vi "TIS_Camera_Polarimeter.vi"() -> ()   [LabVIEW 2025]
panel:
  in  "Degree Sampling":dbl=1.0
  in  "Calibrate QWP":bool
  in  "N Angles":i16=8 min=8 max=200 step=2
  in  "Measure Stokes":bool
  in  "Tab Control":T1(tab)
  in  "ICImagingControl":refnum<k7>(container)
  out "Snapped Image":T2(plugin-control)
  in  "Connect Camera":bool
  in  "Live":bool
  in  "Camera Properties":bool
  out "Camera Ready":bool
  in  "Grab Image":bool
  in  "Stop All":bool
  out "Motor Ready":bool
  in  "Backward":bool
  in  "Forward":bool
  in  "Motor Name":string="0"
  in  "Encoder Steps/º":i32=398
  in  "Jog Angle (º)":dbl=22.5 format="%#_13g"
  in  "VISA Rotatory Motor":refnum<visa-resource-name>="COM4"
  in  "Connect Motor":bool
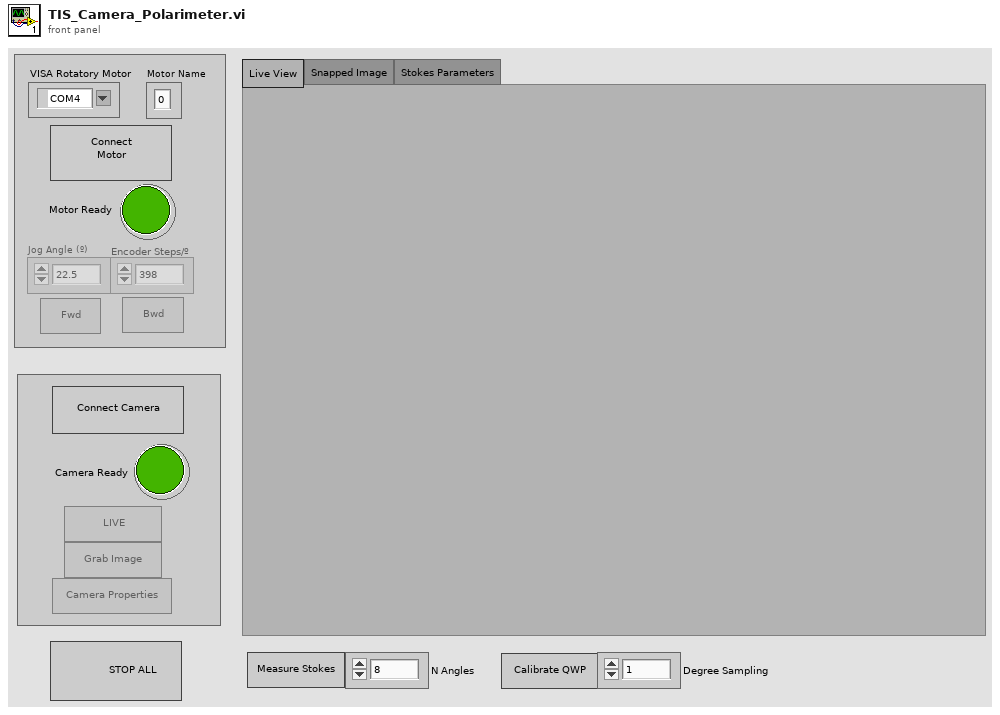
[diagram p1: front panel]
types:
  T1 = enum32{"Live View", "Snapped Image", "Stokes Parameters"}
  T2 = typedef "IMAQ Image.ctl" = refnum<image>
  T3 = typedef "Image Type" = u32
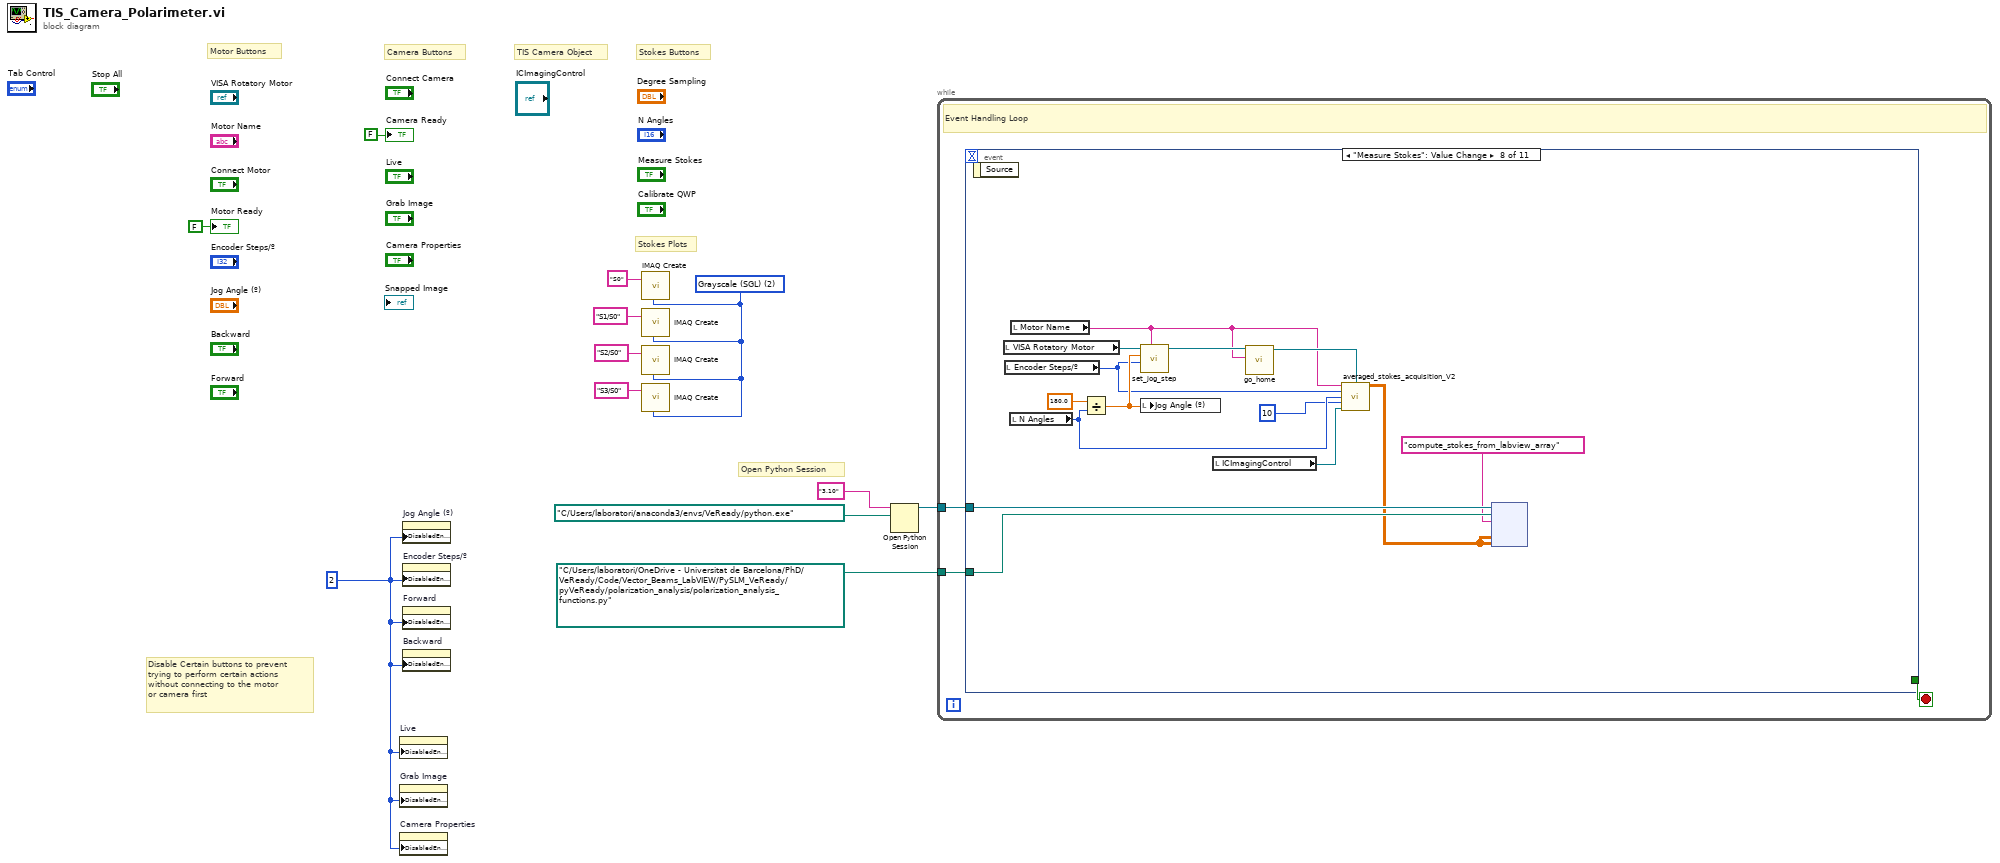
[diagram p0: block diagram]
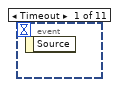
[diagram p2: hidden frame]
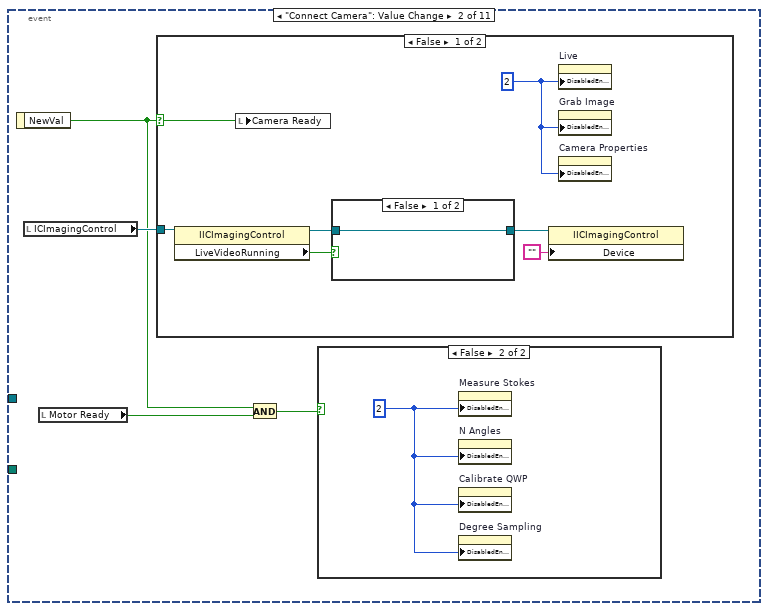
[diagram p3: hidden frame]
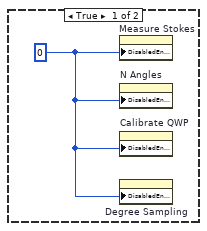
[diagram p4: hidden frame]
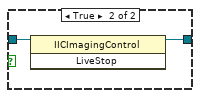
[diagram p5: hidden frame]
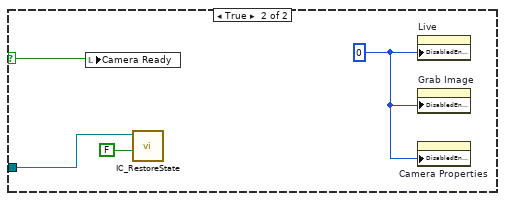
[diagram p6: hidden frame]
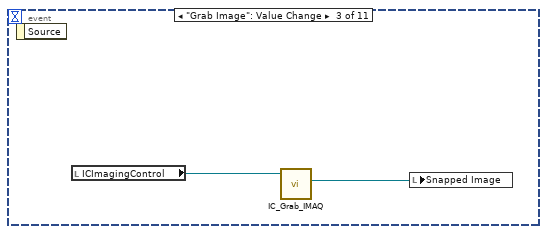
[diagram p7: hidden frame]
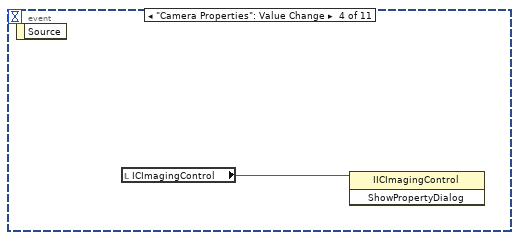
[diagram p8: hidden frame]
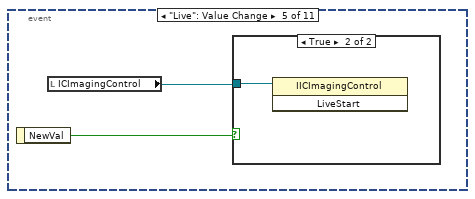
[diagram p9: hidden frame]
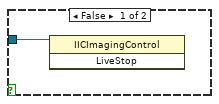
[diagram p10: hidden frame]
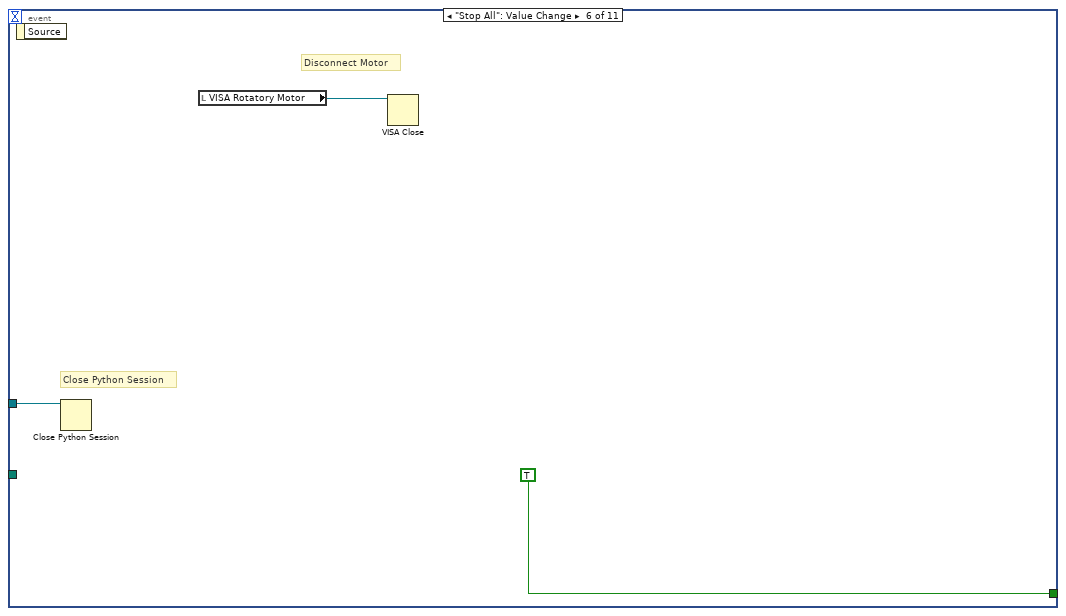
[diagram p11: hidden frame]
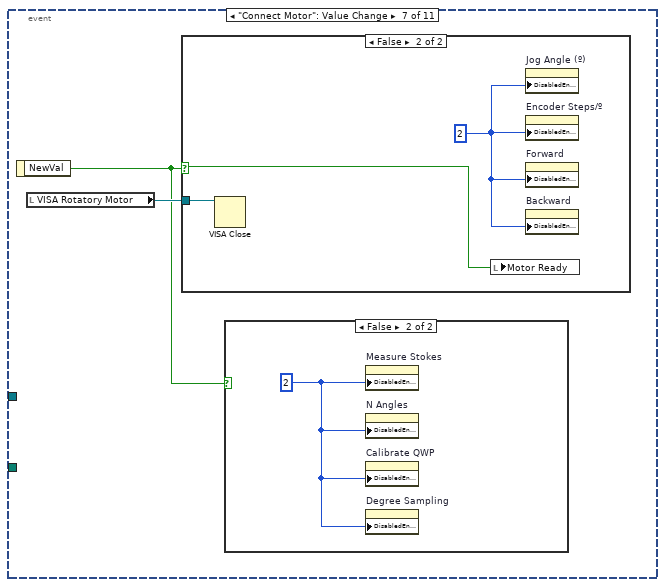
[diagram p12: hidden frame]
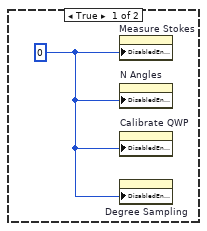
[diagram p13: hidden frame]
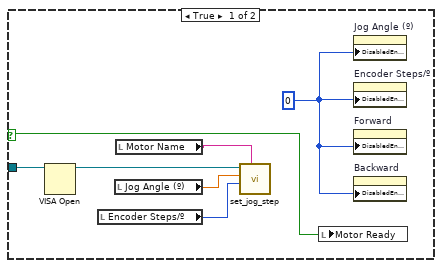
[diagram p14: hidden frame]
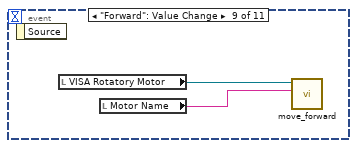
[diagram p15: hidden frame]
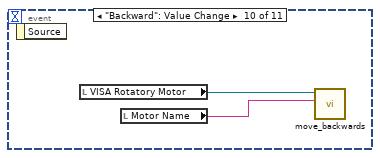
[diagram p16: hidden frame]
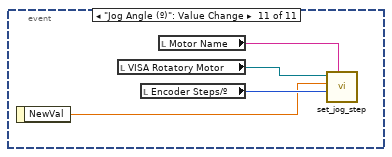
[diagram p17: hidden frame]
diagram:
  w1 = T3 2 items=["Grayscale (U8)", "Grayscale (I16)", "Grayscale (SGL)", "Complex (CSG)", "RGB (U32)", "HSL (U32)", "RGB (U64)", "Grayscale (U16)"] ("Image Type")
  w8 = 2
  # "Stokes Plots"
  # "Stokes Buttons"
  # "TIS Camera Object"
  # "Camera Buttons"
  # "Disable Certain buttons to prevent\ntrying to perform certain actions\nwithout connecting to the motor\nor camera first"
  # "Open Python Session"
  # "Motor Buttons"
  n1 = property on="Live" class="Bool (strict)"("DisabledEnum"=w8) -> ()  [unwired: 2 in, 2 out]
  n2 = property on="Grab Image" class="Bool (strict)"("DisabledEnum"=w8) -> ()  [unwired: 2 in, 2 out]
  n3 = property on="Camera Properties" class="Bool (strict)"("DisabledEnum"=w8) -> ()  [unwired: 2 in, 2 out]
  n4 = property on="Jog Angle (º)" class="DigNum (strict)"("DisabledEnum"=w8) -> ()  [unwired: 2 in, 2 out]
  n5 = property on="Encoder Steps/º" class="DigNum (strict)"("DisabledEnum"=w8) -> ()  [unwired: 2 in, 2 out]
  n6 = property on="Forward" class="Bool"("DisabledEnum"=w8) -> ()  [unwired: 2 in, 2 out]
  n7 = property on="Backward" class="Bool"("DisabledEnum"=w8) -> ()  [unwired: 2 in, 2 out]
  n8 = call "IMAQ Create"("Image Name"="S0", "Image Type"=w1) -> ()  [unwired: 3 in, 2 out]
  n9 = call "IMAQ Create"("Image Name"="S1/S0", "Image Type"=w1) -> ()  [unwired: 3 in, 2 out]
  n10 = call "IMAQ Create"("Image Name"="S2/S0", "Image Type"=w1) -> ()  [unwired: 3 in, 2 out]
  n11 = call "IMAQ Create"("Image Name"="S3/S0", "Image Type"=w1) -> ()  [unwired: 3 in, 2 out]
  n12 = Open Python Session(python version="3.10" ("Python version"), python path=path "C:/Users/laboratori/anaconda3/envs/VeReady/python.exe" ("Python path")) -> (session out=w7:refnum<k35>)  [unwired: 1 in, 1 out]
  n13 = while {
    tunnel: w7 -> [w14]
    tunnel: path "C:/Users/laboratori/OneDrive - Universitat de Barcelona/PhD/VeReady/Code/Vector_Beams_LabVIEW/PySLM_VeReady/pyVeReady/polarization_analysis/polarization_analysis_functions.py" ("module path") -> [w13]
    stop <- w15 stop-if-true
    # "Event Handling Loop"
    n14 = event shown="[7] \"Measure Stokes\": Value Change" {
      selector: _ -> [_ _ _ _ _ _ _ _ _ _ _]
      dyn-events: _ -> [_ _ _ _ _ _ _ _ _ _ _]
      timeout: _ -> [_ _ _ _ _ _ _ _ _ _ _]
      tunnel: [_ _ _ _ _ TRUE _ _ _ _ _] -> w15
      tunnel: w14 -> [_ _ _ _ _ w43 _ w63 _ _ _]
      tunnel: w13 -> [_ _ _ _ _ _ _ w62 _ _ _]
      event Timeout {
        n15 = event-data() -> ()  [unwired: 1 in, 1 out]
      }
      event "Connect Camera": Value Change {
        n16 = event-data() -> ("NewVal"=w17:bool)  [unwired: 1 in]
        n17 = local read "ICImagingControl"() -> (w19:refnum<k7>)
        n18 = local read "Motor Ready"() -> (w16:bool)
        n19 = case shown="False" w17 {
          selector: w17 -> [w22 w32]
          tunnel: w19 -> [w28 w35]
          frame False {
            w23 = 2
            n20 = property class="IICImagingControl"(reference=w28) -> (reference out=w27:refnum<k7>, "LiveVideoRunning"=w26:bool)  [unwired: 1 in, 1 out]
            n21 = local write "Camera Ready"(w22) -> ()
            n22 = case shown="False" w26 {
              tunnel: [w29 w31] -> w25
              tunnel: w27 -> [w29 w30]
              frame False {
              }
              frame True {
                n23 = invoke class="IICImagingControl" method="LiveStop"(reference=w30) -> (reference out=w31:refnum<k7>)  [unwired: 2 in, 2 out]
              }
            }
            n24 = property class="IICImagingControl"(reference=w25, "Device"="") -> ()  [unwired: 1 in, 2 out]
            n25 = property on="Live" class="Bool (strict)"("DisabledEnum"=w23) -> ()  [unwired: 2 in, 2 out]
            n26 = property on="Grab Image" class="Bool (strict)"("DisabledEnum"=w23) -> ()  [unwired: 2 in, 2 out]
            n27 = property on="Camera Properties" class="Bool (strict)"("DisabledEnum"=w23) -> ()  [unwired: 2 in, 2 out]
          }
          frame True {
            w33 = 0
            n28 = local write "Camera Ready"(w32) -> ()
            n29 = call <userlib>:"IC_RestoreState.vi"("Color"=FALSE, "ICImagingControl"=w35) -> ()  [unwired: 2 in, 2 out]
            n30 = property on="Live" class="Bool (strict)"("DisabledEnum"=w33) -> ()  [unwired: 2 in, 2 out]
            n31 = property on="Grab Image" class="Bool (strict)"("DisabledEnum"=w33) -> ()  [unwired: 2 in, 2 out]
            n32 = property on="Camera Properties" class="Bool (strict)"("DisabledEnum"=w33) -> ()  [unwired: 2 in, 2 out]
          }
        }
        n33 = And(x=w17, y=w16) -> (x .and. y?=w18:bool)
        n34 = case shown="False" w18 {
          frame True {
            w20 = 0
            n35 = property on="Measure Stokes" class="Bool (strict)"("DisabledEnum"=w20) -> ()  [unwired: 2 in, 2 out]
            n36 = property on="N Angles" class="DigNum (strict)"("DisabledEnum"=w20) -> ()  [unwired: 2 in, 2 out]
            n37 = property on="Calibrate QWP" class="Bool (strict)"("DisabledEnum"=w20) -> ()  [unwired: 2 in, 2 out]
            n38 = property on="Degree Sampling" class="DigNum (strict)"("DisabledEnum"=w20) -> ()  [unwired: 2 in, 2 out]
          }
          frame False {
            w21 = 2
            n39 = property on="Measure Stokes" class="Bool (strict)"("DisabledEnum"=w21) -> ()  [unwired: 2 in, 2 out]
            n40 = property on="N Angles" class="DigNum (strict)"("DisabledEnum"=w21) -> ()  [unwired: 2 in, 2 out]
            n41 = property on="Calibrate QWP" class="Bool (strict)"("DisabledEnum"=w21) -> ()  [unwired: 2 in, 2 out]
            n42 = property on="Degree Sampling" class="DigNum (strict)"("DisabledEnum"=w21) -> ()  [unwired: 2 in, 2 out]
          }
        }
      }
      event "Grab Image": Value Change {
        n43 = event-data() -> ()  [unwired: 1 in, 1 out]
        n44 = local read "ICImagingControl"() -> (w37:refnum<k7>)
        n45 = call <userlib>:"IC_Grab_IMAQ.vi"("ICImagingControl In"=w37) -> ("Image Out"=w36:T2)  [unwired: 2 in, 3 out]
        n46 = local write "Snapped Image"(w36) -> ()
      }
      event "Camera Properties": Value Change {
        n47 = event-data() -> ()  [unwired: 1 in, 1 out]
        n48 = local read "ICImagingControl"() -> (w38:refnum<k7>)
        n49 = invoke class="IICImagingControl" method="ShowPropertyDialog"(reference=w38) -> ()  [unwired: 2 in, 3 out]
      }
      event "Live": Value Change {
        n50 = event-data() -> ("NewVal"=w39:bool)  [unwired: 1 in]
        n51 = local read "ICImagingControl"() -> (w40:refnum<k7>)
        n52 = case shown="True" w39 {
          tunnel: w40 -> [w41 w42]
          frame False {
            n53 = invoke class="IICImagingControl" method="LiveStop"(reference=w41) -> ()  [unwired: 2 in, 3 out]
          }
          frame True {
            n54 = invoke class="IICImagingControl" method="LiveStart"(reference=w42) -> ()  [unwired: 2 in, 3 out]
          }
        }
      }
      event "Stop All": Value Change {
        # "Close Python Session"
        # "Disconnect Motor"
        n55 = event-data() -> ()  [unwired: 1 in, 1 out]
        n56 = Close Python Session(session in=w43) -> ()  [unwired: 1 in, 1 out]
        n57 = local read "VISA Rotatory Motor"() -> (w44:refnum<visa-resource-name>)
        n58 = VISA Close(VISA resource name=w44) -> ()  [unwired: 1 in, 1 out]
      }
      event "Connect Motor": Value Change {
        n59 = event-data() -> ("NewVal"=w46:bool)  [unwired: 1 in]
        n60 = local read "VISA Rotatory Motor"() -> (w47:refnum<visa-resource-name>)
        n61 = case shown="False" w46 {
          selector: w46 -> [w55 w58]
          tunnel: w47 -> [w56 w59]
          frame True {
            w54 = 0
            n62 = VISA Open(VISA resource name=w56) -> (VISA resource name=w53:refnum<visa-resource-name>)  [unwired: 4 in, 1 out]
            n63 = local read "Encoder Steps/º"() -> (w51:i32)
            n64 = local read "Jog Angle (º)"() -> (w52:dbl)
            n65 = local read "Motor Name"() -> (w50:string)
            n66 = call "set_jog_step.vi"("Motor \"Name\""=w50, "Encoder Pulses per Degree"=w51, "Degrees"=w52, "VISA resource name"=w53) -> ()  [unwired: 5 in, 2 out]
            n67 = local write "Motor Ready"(w55) -> ()
            n68 = property on="Jog Angle (º)" class="DigNum (strict)"("DisabledEnum"=w54) -> ()  [unwired: 2 in, 2 out]
            n69 = property on="Encoder Steps/º" class="DigNum (strict)"("DisabledEnum"=w54) -> ()  [unwired: 2 in, 2 out]
            n70 = property on="Forward" class="Bool"("DisabledEnum"=w54) -> ()  [unwired: 2 in, 2 out]
            n71 = property on="Backward" class="Bool"("DisabledEnum"=w54) -> ()  [unwired: 2 in, 2 out]
          }
          frame False {
            w57 = 2
            n72 = VISA Close(VISA resource name=w59) -> ()  [unwired: 1 in, 1 out]
            n73 = local write "Motor Ready"(w58) -> ()
            n74 = property on="Jog Angle (º)" class="DigNum (strict)"("DisabledEnum"=w57) -> ()  [unwired: 2 in, 2 out]
            n75 = property on="Encoder Steps/º" class="DigNum (strict)"("DisabledEnum"=w57) -> ()  [unwired: 2 in, 2 out]
            n76 = property on="Forward" class="Bool"("DisabledEnum"=w57) -> ()  [unwired: 2 in, 2 out]
            n77 = property on="Backward" class="Bool"("DisabledEnum"=w57) -> ()  [unwired: 2 in, 2 out]
          }
        }
        n78 = case shown="False" w46 {
          frame True {
            w48 = 0
            n79 = property on="Measure Stokes" class="Bool (strict)"("DisabledEnum"=w48) -> ()  [unwired: 2 in, 2 out]
            n80 = property on="N Angles" class="DigNum (strict)"("DisabledEnum"=w48) -> ()  [unwired: 2 in, 2 out]
            n81 = property on="Calibrate QWP" class="Bool (strict)"("DisabledEnum"=w48) -> ()  [unwired: 2 in, 2 out]
            n82 = property on="Degree Sampling" class="DigNum (strict)"("DisabledEnum"=w48) -> ()  [unwired: 2 in, 2 out]
          }
          frame False {
            w49 = 2
            n83 = property on="Measure Stokes" class="Bool (strict)"("DisabledEnum"=w49) -> ()  [unwired: 2 in, 2 out]
            n84 = property on="N Angles" class="DigNum (strict)"("DisabledEnum"=w49) -> ()  [unwired: 2 in, 2 out]
            n85 = property on="Calibrate QWP" class="Bool (strict)"("DisabledEnum"=w49) -> ()  [unwired: 2 in, 2 out]
            n86 = property on="Degree Sampling" class="DigNum (strict)"("DisabledEnum"=w49) -> ()  [unwired: 2 in, 2 out]
          }
        }
      }
      event "Measure Stokes": Value Change {
        n87 = event-data() -> ()  [unwired: 1 in, 1 out]
        n88 = local read "VISA Rotatory Motor"() -> (w73:refnum<visa-resource-name>)
        n89 = local read "Encoder Steps/º"() -> (w66:i32)
        n90 = local read "N Angles"() -> (w67:i16)
        n91 = local read "Motor Name"() -> (w68:string)
        n92 = Divide(x=180.0, y=w67) -> (x/y=w71:dbl)
        n93 = call "set_jog_step.vi"("Motor \"Name\""=w68, "Encoder Pulses per Degree"=w66, "Degrees"=w71, "VISA resource name"=w73) -> ("VISA resource name out"=w70:refnum<visa-resource-name>)  [unwired: 5 in, 1 out]
        n94 = local write "Jog Angle (º)"(w71) -> ()
        n95 = local read "ICImagingControl"() -> (w64:refnum<k7>)
        n96 = call "go_home.vi"("Motor \"Name\""=w68, "VISA resource name"=w70) -> ("VISA resource name out"=w69:refnum<visa-resource-name>)  [unwired: 8 in, 1 out]
        n97 = call "averaged_stokes_acquisition_V2.vi"("Motor \"Name\""=w68, "VISA resource name"=w69, "Encoder Pulses per Degree"=w66, "Number of Angles"=w67, "Number of Measures"=10, "ICImagingControl In"=w64) -> ("Polarimetric Images 3D Array"=w60:dbl[][][])  [unwired: 9 in]
        n98 = node(w63, w62, "compute_stokes_from_labview_array" ("function name"), w60, w60) -> ()  [unwired: 3 in, 4 out]
      }
      event "Forward": Value Change {
        n99 = event-data() -> ()  [unwired: 1 in, 1 out]
        n100 = local read "VISA Rotatory Motor"() -> (w75:refnum<visa-resource-name>)
        n101 = local read "Motor Name"() -> (w74:string)
        n102 = call "move_forward.vi"("Motor \"Name\""=w74, "VISA resource name"=w75) -> ()  [unwired: 8 in, 2 out]
      }
      event "Backward": Value Change {
        n103 = event-data() -> ()  [unwired: 1 in, 1 out]
        n104 = local read "VISA Rotatory Motor"() -> (w77:refnum<visa-resource-name>)
        n105 = local read "Motor Name"() -> (w76:string)
        n106 = call "move_backwards.vi"("Motor \"Name\""=w76, "VISA resource name"=w77) -> ()  [unwired: 8 in, 2 out]
      }
      event "Jog Angle (º)": Value Change {
        n107 = event-data() -> ("NewVal"=w79:dbl)  [unwired: 1 in]
        n108 = local read "VISA Rotatory Motor"() -> (w80:refnum<visa-resource-name>)
        n109 = local read "Encoder Steps/º"() -> (w81:i32)
        n110 = local read "Motor Name"() -> (w78:string)
        n111 = call "set_jog_step.vi"("Motor \"Name\""=w78, "Encoder Pulses per Degree"=w81, "Degrees"=w79, "VISA resource name"=w80) -> ()  [unwired: 5 in, 2 out]
      }
    }
  }
  "Motor Ready" <- FALSE ("Motor Ready")
  "Camera Ready" <- FALSE ("Camera Ready")
